vi "Close Caller.vi"(8 "error in (no error)":errorcluster, 10 "Caller":T1, 11 "Open Close Logic Simple Table in":refnum<class "Open Close Logic Simple Table.lvclass">) -> (0 "error out":errorcluster, 2 "Close Nested":T1[](array[typedef]), 3 "Open Close Logic Simple Table out":refnum<class "Open Close Logic Simple Table.lvclass">)   [LabVIEW 2020, in "Open Close Logic Simple Table.lvlib" / "Open Close Logic Simple Table.lvclass"]
uses:
  Open Close Logic Simple Table.lvclass
  Form ID.ctl
  Open Close Logic Simple Table.lvclass/Open Close Logic Simple Table.ctl
  <userlib>/_OpenG.lib/array/array.llb/Search 1D Array (Variant)__ogtk.vi
  <userlib>/_OpenG.lib/array/array.llb/Delete Elements from 1D Array (Variant)__ogtk.vi
  Form Server Interfaces.lvlib
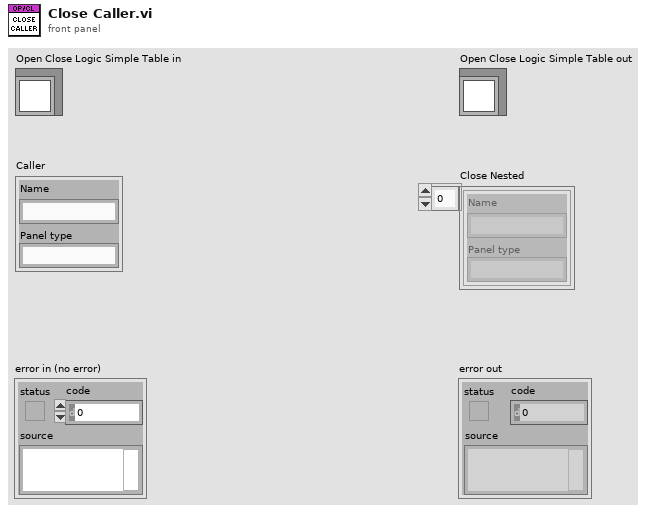
[diagram p1: front panel]
types:
  T1 = typedef "Form Server Interfaces.lvlib/Form ID.ctl" = cluster{"Name":string, "Panel type":string}
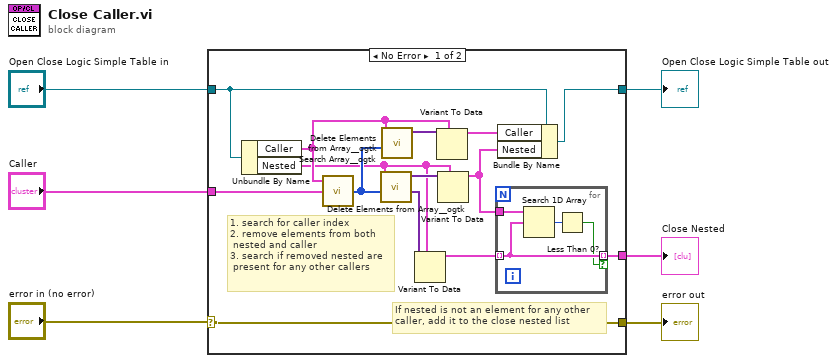
[diagram p0: block diagram]
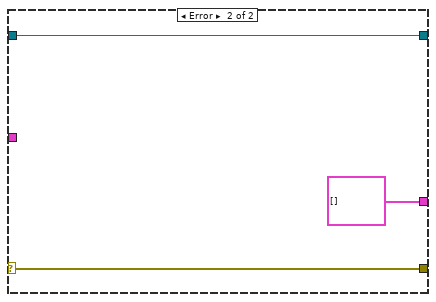
[diagram p2: hidden frame]
diagram:
  n1 = case shown="No Error" "error in (no error)" {
    selector: "error in (no error)" -> [w20 w27]
    tunnel: [w20 w27] -> w5
    tunnel: "Open Close Logic Simple Table in" -> [w13 w26]
    tunnel: [w12 w26] -> w3
    tunnel: "Caller" -> [w19 _]
    tunnel: [w17 T1[] []] -> w1
    frame No Error {
      # "1. search for caller index\n2. remove elements from both\n nested and caller\n3. search if removed nested are\n present for any other callers"
      # "If nested is not an element for any other\ncaller, add it to the close nested list"
      n2 = Unbundle By Name(w13) -> ("Caller"=w10:T1[], "Nested"=w7:T1[])
      n3 = call-poly <userlib>:"Search Array__ogtk.vi"("Array"=w10, "Element Data"=w19) -> ("Indices of Elements"=w16:i32[])  [unwired: 7 in]
      n4 = call-poly <userlib>:"Delete Elements from Array__ogtk.vi"("indices"=w16, "array"=w7) -> ("deleted elements"=w8:variant[], "array w/ subset deleted"=w14:variant[])  [unwired: 8 in]
      n5 = call-poly <userlib>:"Delete Elements from Array__ogtk.vi"("indices"=w16, "array"=w10) -> ("array w/ subset deleted"=w15:variant[])  [unwired: 8 in, 1 out]
      n6 = Variant To Data(type=w7, Variant=w8) -> (data=w18:T1[])  [unwired: 1 in, 1 out]
      n7 = Variant To Data(type=w10, Variant=w15) -> (data=w11:T1[])  [unwired: 1 in, 1 out]
      n8 = Variant To Data(type=w7, Variant=w14) -> (data=w9:T1[])  [unwired: 1 in, 1 out]
      n9 = for {
        tunnel: w18 -> [w23] mode=indexing
        tunnel: w9 -> [w24]
        tunnel: [w23] -> w17 mode=indexing if=w21
        n10 = Search 1D Array(1D array=w24, element=w23) -> (index of element=w22:i32)  [unwired: 1 in]
        n11 = Less Than 0?(x=w22) -> (x < 0?=w21:bool)
      }
      n12 = Bundle By Name(cluster=w13, "Caller"=w11, "Nested"=w9) -> (w12:refnum<class "Open Close Logic Simple Table.lvclass">)
    }
    frame Error {
    }
  }
  "error out" <- w5
  "Open Close Logic Simple Table out" <- w3
  "Close Nested" <- w1
